vi "create_plot_surface.vi"(6 "plot ID":i32, 7 "color matrix":dbl[][](array[numeric]), 8 "z matrix":dbl[][](array[numeric]), 9 "y vector":dbl[](array[numeric]), 10 "x vector":dbl[](array[numeric]), 11 "plots in":refnum<class "Base Datatype.lvclass">[](array[class])) -> (3 "plots out":refnum<class "Base Datatype.lvclass">[](array[class]))   [LabVIEW 2020, in "3DPC_SurfacePlot.xctl"]
doc: "Plots a surface in terms of x, y, and z points. This VI has two 1D arrays and one 2D array that specify each point on the plot."
uses:
  <vilib>/Native 3D Graph/xcontrol/3DPC_SurfacePlot.xctl
  <vilib>/Native 3D Graph/classes/Base Datatype.lvclass
  <vilib>/Native 3D Graph/classes/Surface/Surface.lvclass
  e:/builds/penguin/labview/branches/2020/dev/dist/vi.lib/Native 3D Graph/classes/Base Datatype.lvclass
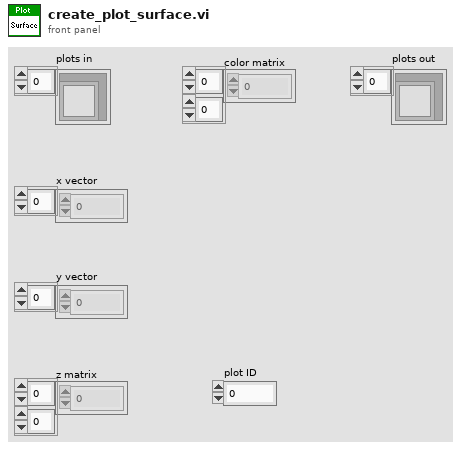
[diagram p1: front panel]
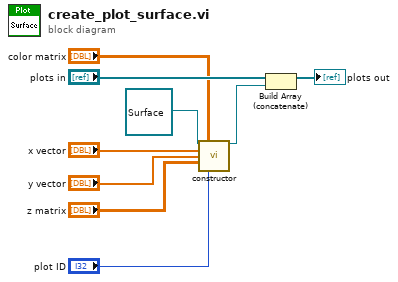
[diagram p0: block diagram]
diagram:
  n1 = call-dynamic "constructor.vi"("Surface in"=refnum<class "Surface.lvclass"> refnum, "Color Matrix"="color matrix", "X vector"="x vector", "Y vector"="y vector", "Z Matrix"="z matrix", "Plot ID"="plot ID") -> ("Surface out"=w2:refnum<class "Surface.lvclass">)  [unwired: 1 in, 8 out]
  n2 = Build Array (concatenate)("plots in", w2) -> (→"plots out":refnum<class "Base Datatype.lvclass">[])
